vi "Preview Sensor.vi"(8 "error in (no error)":errorcluster, 11 "Sensor Model in":refnum<class "Sensor Model.lvclass">) -> (0 "error out":errorcluster, 3 "Sensor Model out":refnum<class "Sensor Model.lvclass">)   [LabVIEW 2013, in "Sensor Model.lvlib" / "Sensor Model.lvclass"]
uses:
  Sensor Model.lvclass
  Sensor Model.lvclass/Sensor Model.ctl
  <vilib>/xml/Load XML File.vi
  <vilib>/xml/Close Reference(Node).vi
  <vilib>/xml/NI_XML.lvlib
  Common/File IO/File IO.lvlib
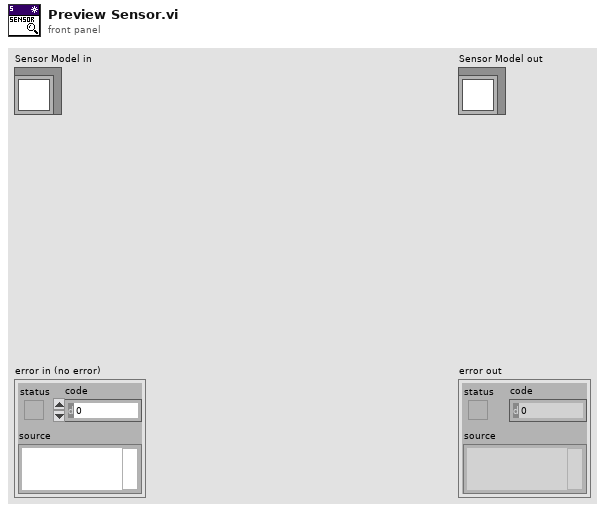
[diagram p1: front panel]
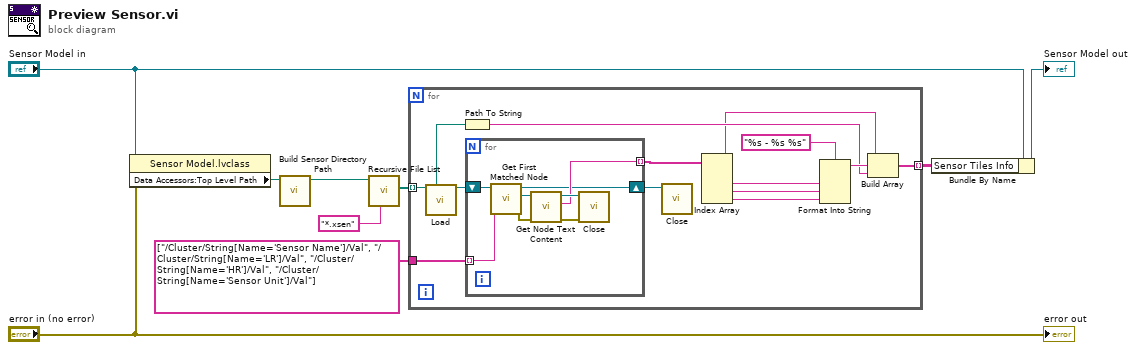
[diagram p0: block diagram]
diagram:
  n1 = property class="Sensor Model.lvclass"(reference="Sensor Model in", error in="error in (no error)") -> ("Data Accessors:Top Level Path"=w9:path)  [unwired: 2 out]
  n2 = call "Build Sensor Directory Path.vi"("Top Level Path"=w9) -> ("Sensor Directory Path"=w7:path)  [unwired: 10 in]
  n3 = call <vilib>:"Recursive File List.vi"("pattern"="*.xsen", "Folder Path"=w7) -> ("All Files in Dir"=w6:path[])  [unwired: 5 in, 4 out]
  n4 = for {
    tunnel: w6 -> [w20] mode=indexing
    tunnel: string[] ["/Cluster/String[Name='Sensor Name']/Val", "/Cluster/String[Name='LR']/Val", "/Cluster/String[Name='HR']/Val", "/Cluster/String[Name='Sensor Unit']/Val"] -> [w21]
    tunnel: [w18] -> w3 mode=indexing
    n5 = call-poly <vilib>:"Load.vi"("path to XML document"=w20) -> ("DOM document out"=w22:refnum<k20>)  [unwired: 12 in, 2 out]
    n6 = Path To String(path=w20) -> (string=w11:string)
    n7 = for {
      shift-right: [w23] -> w19
      shift-left: w22 -> [w30]
      tunnel: w21 -> [w29] mode=indexing
      tunnel: [w26] -> w17 mode=indexing
      n8 = call <vilib>:"Get First Matched Node.vi"("XPath expression"=w29, "node in"=w30) -> ("error out"=w24:errorcluster, "node result"=w28:refnum<k20>, "node out"=w23:refnum<k20>)  [unwired: 7 in]
      n9 = call <vilib>:"Get Node Text Content.vi"("error in (no error)"=w24, "node in"=w28) -> ("error out"=w25:errorcluster, "node text"=w26:string, "node out"=w27:refnum<k20>)  [unwired: 7 in]
      n10 = call-poly <vilib>:"Close.vi"("error in (no error)"=w25, "node"=w27) -> ()  [unwired: 7 in, 1 out]
    }
    n11 = call-poly <vilib>:"Close.vi"("node"=w19) -> ()  [unwired: 8 in, 1 out]
    n12 = Index Array(array=w17) -> (element #1=w10:string, element #2=w15:string, element #3=w14:string, element #4=w13:string)  [unwired: 4 in]
    n13 = Format Into String(format string="%s - %s %s", w15, w14, w13) -> (resulting string=w12:string)  [unwired: 2 in, 1 out]
    n14 = Build Array(w10, w12, w11) -> (w18:string[])
  }
  n15 = Bundle By Name(cluster="Sensor Model in", "Sensor Tiles Info"=w3) -> (→"Sensor Model out":refnum<class "Sensor Model.lvclass">)
  "error out" <- "error in (no error)"
